vi "DFS Data - Set Current Index.vi"(1 "Current Index":i32, 2 "DFS Data In":T1) -> (0 "DFS Data Out":T1)   [LabVIEW 2022 SP3]
doc: "<add documentation here>"
uses:
  DFS Data (cluster).ctl
  DFS Node (cluster).ctl
  DFS Child Node (cluster).ctl
panel:
  # "Development\nControls or indicators that are useful for development or testing, but which are not outputs of the VI."
  # "Input\nInputs to the VI"
  # "Output\nOutputs of the VI"
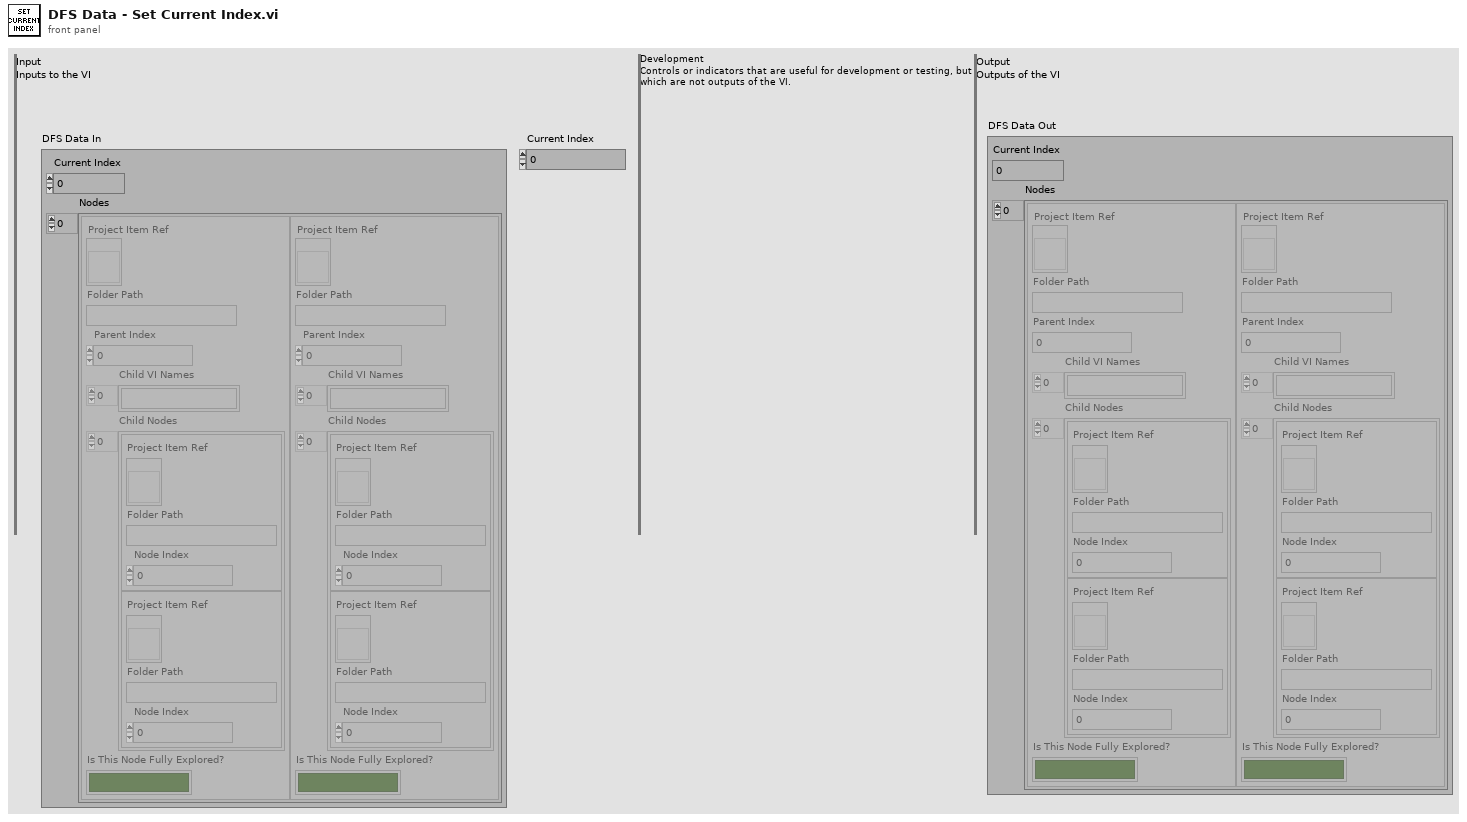
[diagram p1: front panel]
types:
  T1 = typedef "DFS Data (cluster).ctl" = cluster{"Current Index":i32, "Nodes":T2[]}
  T2 = typedef "DFS Node (cluster).ctl" = cluster{"Project Item Ref":refnum<vi>, "Folder Path":string, "Parent Index":i32, "Child VI Names":string[], "Child Nodes":T3[], "Is This Node Fully Explored?":bool}
  T3 = typedef "DFS Child Node (cluster).ctl" = cluster{"Project Item Ref":refnum<vi>, "Folder Path":string, "Node Index":i32}
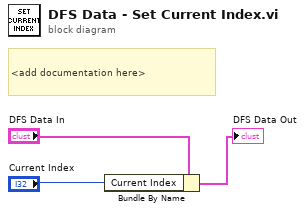
[diagram p0: block diagram]
diagram:
  # "<add documentation here>"
  n1 = Bundle By Name(cluster="DFS Data In", "Current Index"="Current Index") -> (→"DFS Data Out":T1)
